vi "Start Sync.vi"(8 "error in (no error)":errorcluster, 10 "current time":timestamp, 11 "gRPC Server in":refnum<class "OCVTest.lvclass">) -> (0 "error out":errorcluster, 3 "gRPC Server out":refnum<class "OCVTest.lvclass">)   [LabVIEW 2019, in "OCVTest.lvlib" / "OCVTest.lvclass"]
uses:
  OCVTest.lvclass
  OCVTest.lvclass/OCVTest.ctl
  RPC Messages/measurementservice_QueryResponse/measurementservice_QueryResponse_Data.ctl
  RPC Messages/measurementservice_ErrorOut/measurementservice_ErrorOut_Data.ctl
  RPC Messages/measurementservice_OCVRaw/measurementservice_OCVRaw_Data.ctl
  RPC Messages/measurementservice_OCVData/measurementservice_OCVData_Data.ctl
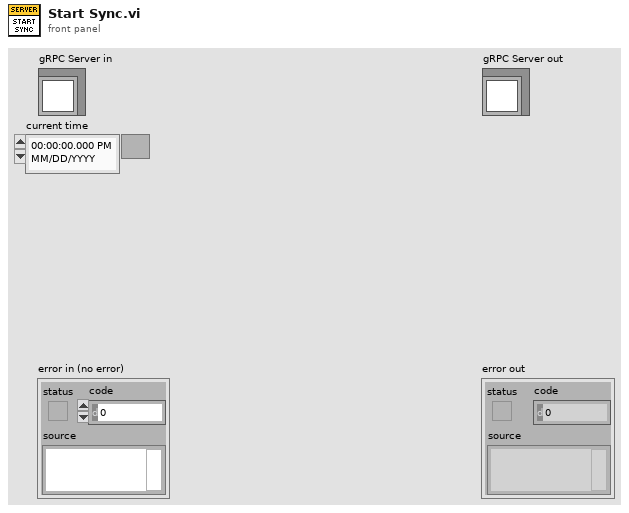
[diagram p1: front panel]
types:
  T1 = typedef "OCVTest.lvlib/OCVTest.lvclass/measurementservice_QueryResponse_Data.ctl" = cluster{"message":string, "status":i32}
  T2 = typedef "OCVTest.lvlib/OCVTest.lvclass/measurementservice_OCVData_Data.ctl" = cluster{"data":T3[]}
  T3 = typedef "OCVTest.lvlib/OCVTest.lvclass/measurementservice_OCVRaw_Data.ctl" = cluster{"battery1voltage":sgl, "battery2voltage":sgl, "battery3voltage":sgl, "battery4voltage":sgl, "battery5voltage":sgl, "battery6voltage":sgl, "battery7voltage":sgl, "battery8voltage":sgl, "battery9voltage":sgl, "battery10voltage":sgl, "battery11voltage":sgl, "battery12voltage":sgl, "battery13voltage":sgl, "battery14voltage":sgl, "battery15voltage":sgl, "battery16voltage":sgl, "battery17voltage":sgl, "battery18voltage":sgl, "battery19voltage":sgl, "battery20voltage":sgl, "battery21voltage":sgl, "battery22voltage":sgl, "battery23voltage":sgl, "battery24voltage":sgl, "error":T4}
  T4 = typedef "OCVTest.lvlib/OCVTest.lvclass/measurementservice_ErrorOut_Data.ctl" = cluster{"errCode":i32, "errMessage":string}
  T5 = typedef "OCVTest.lvlib/OCVTest.lvclass/Server gRPC UEs.ctl" = cluster{"Invoke gRPC UE":refnum<user-event>, "Query gRPC UE":refnum<user-event>, "PerformOCVMeasurement gRPC UE":refnum<user-event>, "PerformACIRMeasurement gRPC UE":refnum<user-event>, "StreamOCVMeasurement gRPC UE":refnum<user-event>, "Register gRPC UE":refnum<user-event>}
  T6 = typedef "OCVTest.lvlib/gprc-lvsupport.lvlib/grpcId.ctl" = u64
  T7 = typedef "OCVTest.lvlib/OCVTest.lvclass/measurementservice_QueryRequest_Data.ctl" = cluster{"query":string}
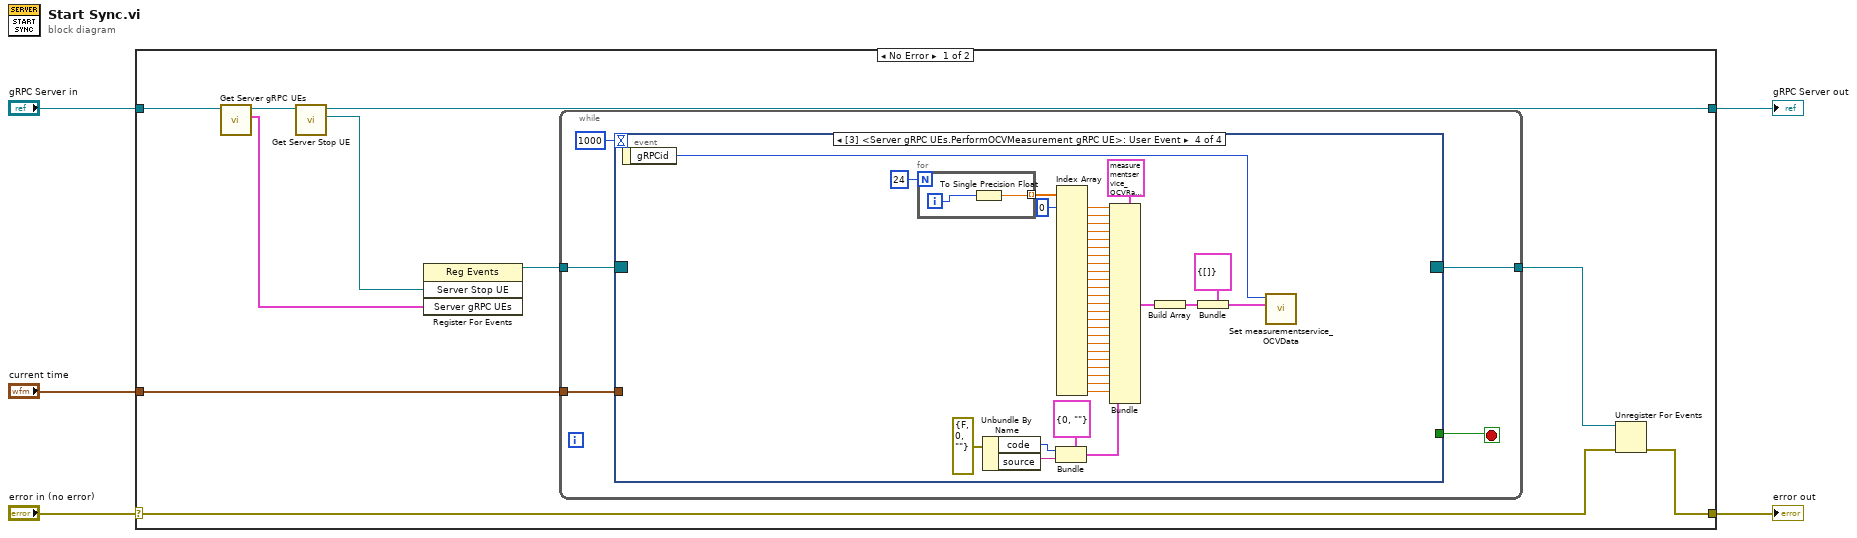
[diagram p0: block diagram]
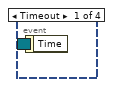
[diagram p2: hidden frame]
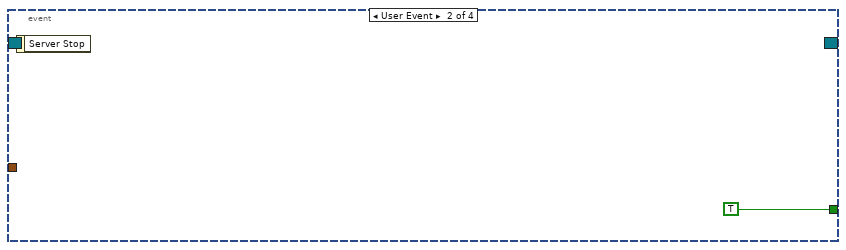
[diagram p3: hidden frame]
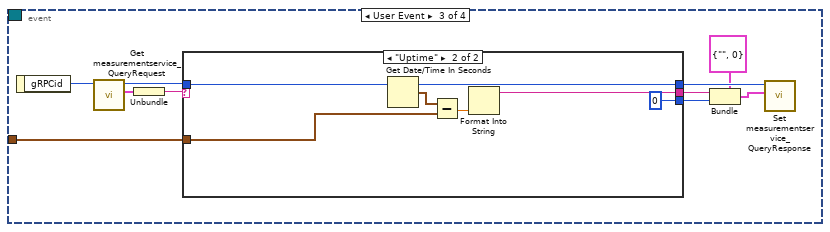
[diagram p4: hidden frame]
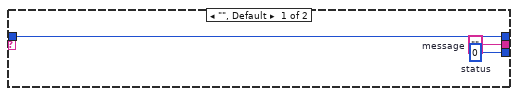
[diagram p5: hidden frame]
diagram:
  n1 = case shown="No Error" "error in (no error)" {
    selector: "error in (no error)" -> [w8 w82]
    tunnel: [w7 w82] -> w4
    tunnel: [w11 w81] -> w2
    tunnel: "gRPC Server in" -> [w15 w81]
    tunnel: "current time" -> [w6 _]
    frame No Error {
      n2 = call "Get Server gRPC UEs.vi"("OOP Server in"=w15) -> ("Server gRPC UEs"=w12:T5, "OOP Server out"=w14:refnum<class "OCVTest.lvclass">)  [unwired: 9 in]
      n3 = call "Get Server Stop UE.vi"("OOP Server in"=w14) -> ("Server Stop UE"=w13:refnum<user-event>, "OOP Server out"=w11:refnum<class "OCVTest.lvclass">)  [unwired: 9 in]
      n4 = register-events(w13, w12) -> (reference out=w10:refnum<event-registration>)  [unwired: 2 in, 1 out]
      n5 = while {
        tunnel: w10 -> [w20]
        tunnel: [w18] -> w9
        tunnel: w6 -> [w16]
        stop <- w19 stop-if-true
        n6 = event "RPC Methods Event Structure" shown="[3] <Server gRPC UEs.PerformOCVMeasurement gRPC UE>: User Event" {
          selector: w20 -> [_ _ _ _]
          dyn-events: [_ _ _ _] -> w18
          timeout: 1000 -> [_ _ _ _]
          tunnel: [_ TRUE _ _] -> w19
          tunnel: w16 -> [_ _ w31 _]
          event Timeout {
            n7 = event-data() -> ()  [unwired: 1 in, 1 out]
          }
          event User Event {
            n8 = event-data() -> ()  [unwired: 1 in, 1 out]
          }
          event User Event {
            n9 = event-data() -> ("gRPCid"=w30:T6)  [unwired: 1 in]
            n10 = call "Get measurementservice_QueryRequest.vi"("gRPCid"=w30) -> ("Message Data"=w28:T7, "gRPCid out"=w29:T6)  [unwired: 8 in, 1 out]
            n11 = Unbundle(w28) -> ("query"=w27:string)
            n12 = case shown="\"Uptime\"" w27 {
              tunnel: w29 -> [w34 w37]
              tunnel: [w34 w37] -> w26
              tunnel: [w33 w38] -> w24
              tunnel: [w32 0 ("status")] -> w23
              tunnel: w31 -> [_ w35]
              frame "", Default {
                w32 = 0  # status
                w33 = ""  # message
              }
              frame "Uptime" {
                n13 = Get Date/Time In Seconds() -> (seconds since 1Jan1904=w40:timestamp)
                n14 = Subtract(x=w40, y=w35) -> (x-y=w39:dbl)
                n15 = Format Into String(w39) -> (resulting string=w38:string)  [unwired: 3 in, 1 out]
              }
            }
            n16 = Bundle(cluster=T1 {"message"="", "status"=0} ("Message Data"), "message"=w24, "status"=w23) -> (w22:T1)
            n17 = call "Set measurementservice_QueryResponse.vi"("Message Data"=w22, "gRPCid"=w26) -> ()  [unwired: 9 in, 1 out]
          }
          event User Event {
            n18 = event-data() -> ("gRPCid"=w42:T6)  [unwired: 1 in]
            n19 = for {
              N: 24 -> [_]
              tunnel: [w80] -> w78 mode=indexing
              i -> [w79]
              n20 = To Single Precision Float(number=w79) -> (single precision float=w80:sgl)
            }
            n21 = Unbundle By Name(errorcluster {"status"=FALSE, "code"=0, "source"=""} ("input cluster")) -> ("code"=w51:i32, "source"=w52:string)
            n22 = Bundle(cluster=T4 {"errCode"=0, "errMessage"=""} ("measurementservice_ErrorOut_Data"), "errCode"=w51, "errMessage"=w52) -> (w53:T4)
            n23 = Index Array(array=w78, index #1=0 ("index")) -> (element #1=w54:sgl, element #2=w55:sgl, element #3=w56:sgl, element #4=w57:sgl, element #5=w58:sgl, element #6=w59:sgl, element #7=w60:sgl, element #8=w61:sgl, element #9=w62:sgl, element #10=w63:sgl, element #11=w64:sgl, element #12=w65:sgl, element #13=w66:sgl, element #14=w67:sgl, element #15=w68:sgl, element #16=w69:sgl, element #17=w70:sgl, element #18=w71:sgl, element #19=w72:sgl, element #20=w73:sgl, element #21=w74:sgl, element #22=w75:sgl, element #23=w76:sgl, element #24=w77:sgl)  [unwired: 23 in]
            n24 = Bundle(cluster=T3 {"battery1voltage"=0.0, "battery2voltage"=0.0, "battery3voltage"=0.0, "battery4voltage"=0.0, "battery5voltage"=0.0, "battery6voltage"=0.0, "battery7voltage"=0.0, "battery8voltage"=0.0, "battery9voltage"=0.0, "battery10voltage"=0.0, "battery11voltage"=0.0, "battery12voltage"=0.0, "battery13voltage"=0.0, "battery14voltage"=0.0, "battery15voltage"=0.0, "battery16voltage"=0.0, "battery17voltage"=0.0, "battery18voltage"=0.0, "battery19voltage"=0.0, "battery20voltage"=0.0, "battery21voltage"=0.0, "battery22voltage"=0.0, "battery23voltage"=0.0, "battery24voltage"=0.0, "error"={"errCode"=0, "errMessage"=""}} ("measurementservice_OCVRaw_Data"), "battery1voltage"=w54, "battery2voltage"=w55, "battery3voltage"=w56, "battery4voltage"=w57, "battery5voltage"=w58, "battery6voltage"=w59, "battery7voltage"=w60, "battery8voltage"=w61, "battery9voltage"=w62, "battery10voltage"=w63, "battery11voltage"=w64, "battery12voltage"=w65, "battery13voltage"=w66, "battery14voltage"=w67, "battery15voltage"=w68, "battery16voltage"=w69, "battery17voltage"=w70, "battery18voltage"=w71, "battery19voltage"=w72, "battery20voltage"=w73, "battery21voltage"=w74, "battery22voltage"=w75, "battery23voltage"=w76, "battery24voltage"=w77, "error"=w53) -> (w46:T3)
            n25 = Build Array(w46) -> (w44:T3[])
            n26 = Bundle(cluster=T2 {"data"=[]} ("Message Data"), "data"=w44) -> (w43:T2)
            n27 = call "Set measurementservice_OCVData.vi"("Message Data"=w43, "gRPCid"=w42) -> ()  [unwired: 9 in, 1 out]
          }
        }
      }
      n28 = Unregister For Events(event registration refnum=w9, error in=w8) -> (error out=w7:errorcluster)
    }
    frame Error {
    }
  }
  "error out" <- w4
  "gRPC Server out" <- w2
